vi "Config Reference.vi"(4 "Loss Percent (off)":bool, 5 "Capacitance Mode (off)":bool, 6 "Capacitance Percent (off)":bool, 7 "Loss Mode (off)":bool, 8 "error in":errorcluster, 9 "Loss Point (0 jpF)":dbl min=-99999999.0 max=99999999.0 format="%#_10f", 10 "Capacitance Point (0 pF)":dbl min=-99999999.0 max=99999999.0 format="%#_10f", 11 "VISA resource name":refnum<visa-resource-name>) -> (0 "error out":errorcluster, 3 "VISA resource name out":refnum<visa-resource-name>)   [LabVIEW 2014, in "Andeen-Hagerling 2700.lvlib"]
doc: "This VI provides the ability to manually entering the capacitance and loss Reference points, and change\nbridge mode between “Absolute result mode” and “Reference result mode.” Also provides the ability to select wether Reference result mode measurement values are reported as simple or percent differences."
uses:
  Andeen-Hagerling 2700.lvlib
panel:
  # "Reference Parameters"
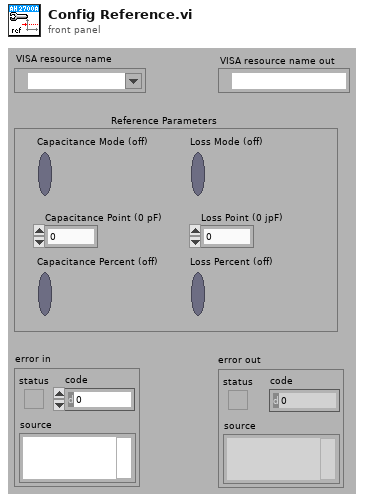
[diagram p1: front panel]
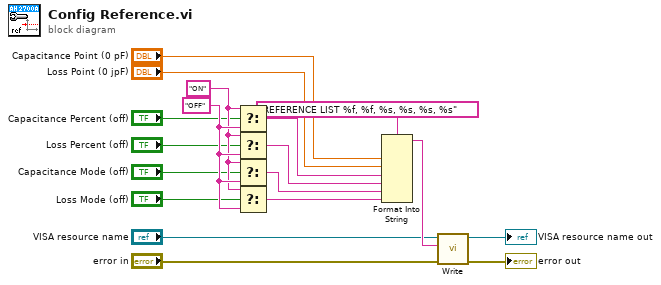
[diagram p0: block diagram]
diagram:
  w18 = "OFF"
  w17 = "ON"
  n1 = Select(t=w17, s="Capacitance Percent (off)", f=w18) -> (s? t:f=w4:string)
  n2 = Select(t=w17, s="Loss Percent (off)", f=w18) -> (s? t:f=w5:string)
  n3 = Select(t=w17, s="Capacitance Mode (off)", f=w18) -> (s? t:f=w16:string)
  n4 = Select(t=w17, s="Loss Mode (off)", f=w18) -> (s? t:f=w15:string)
  n5 = Format Into String(format string="REFERENCE LIST %f, %f, %s, %s, %s, %s", "Capacitance Point (0 pF)", "Loss Point (0 jpF)", w4, w5, w16, w15) -> (resulting string=w14:string)  [unwired: 2 in, 1 out]
  n6 = call "Write.vi"("error in"="error in", "command"=w14, "VISA resource name"="VISA resource name") -> ("error out"=→"error out":errorcluster, "VISA resource name out"=→"VISA resource name out":refnum<visa-resource-name>)  [unwired: 7 in]
